vi "Mask From Contour.vi"(0 "Contour":T1, 1 "Size":T2, 5 "error in (no error)":errorcluster) -> (14 "image out":refnum<class "MSC Image.lvclass">, 15 "contourAreaPixel":dbl, 16 "contourLengthPixel":dbl, 17 "Bounding Box":T1, 19 "error out":errorcluster)   [LabVIEW 2016, in "MSC Image.lvclass"]
doc: "Calculates a mask image from a contour. Each pixel within the contour is marked."
uses:
  MSC Image.lvclass
  Dependencies/x86/MSC I Process32.dll
  controls/Image Type.ctl
  controls/Contour.ctl
  controls/Size.ctl
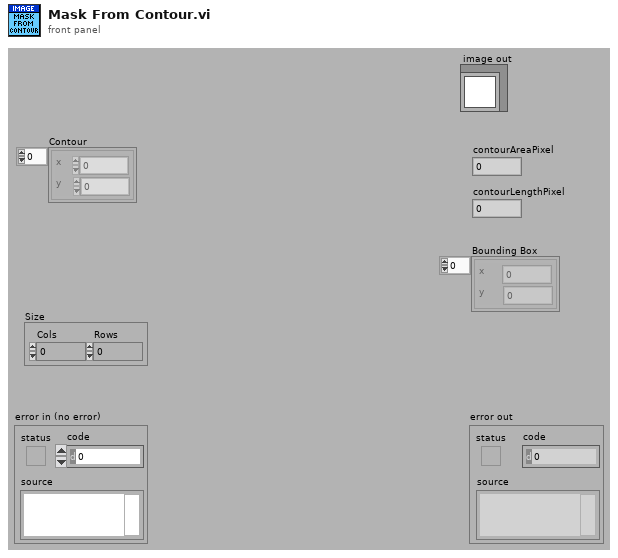
[diagram p1: front panel]
types:
  T1 = typedef "MSC Image.lvclass/Contour.ctl" = cluster{"x":i16, "y":i16}[]
  T2 = typedef "MSC Image.lvclass/Size.ctl" = cluster{"Cols":i32, "Rows":i32}
  T3 = typedef "MSC Image.lvclass/Image Type.ctl" = i32
  T4 = typedef "Image.ctl" = cluster{"Pointer":u64, "Size":T5, "Image Type":T6, "Time Stamp":timestamp, "Variant":variant}
  T5 = typedef "Size.ctl" = cluster{"Cols":i32, "Rows":i32}
  T6 = typedef "Image Type.ctl" = i32
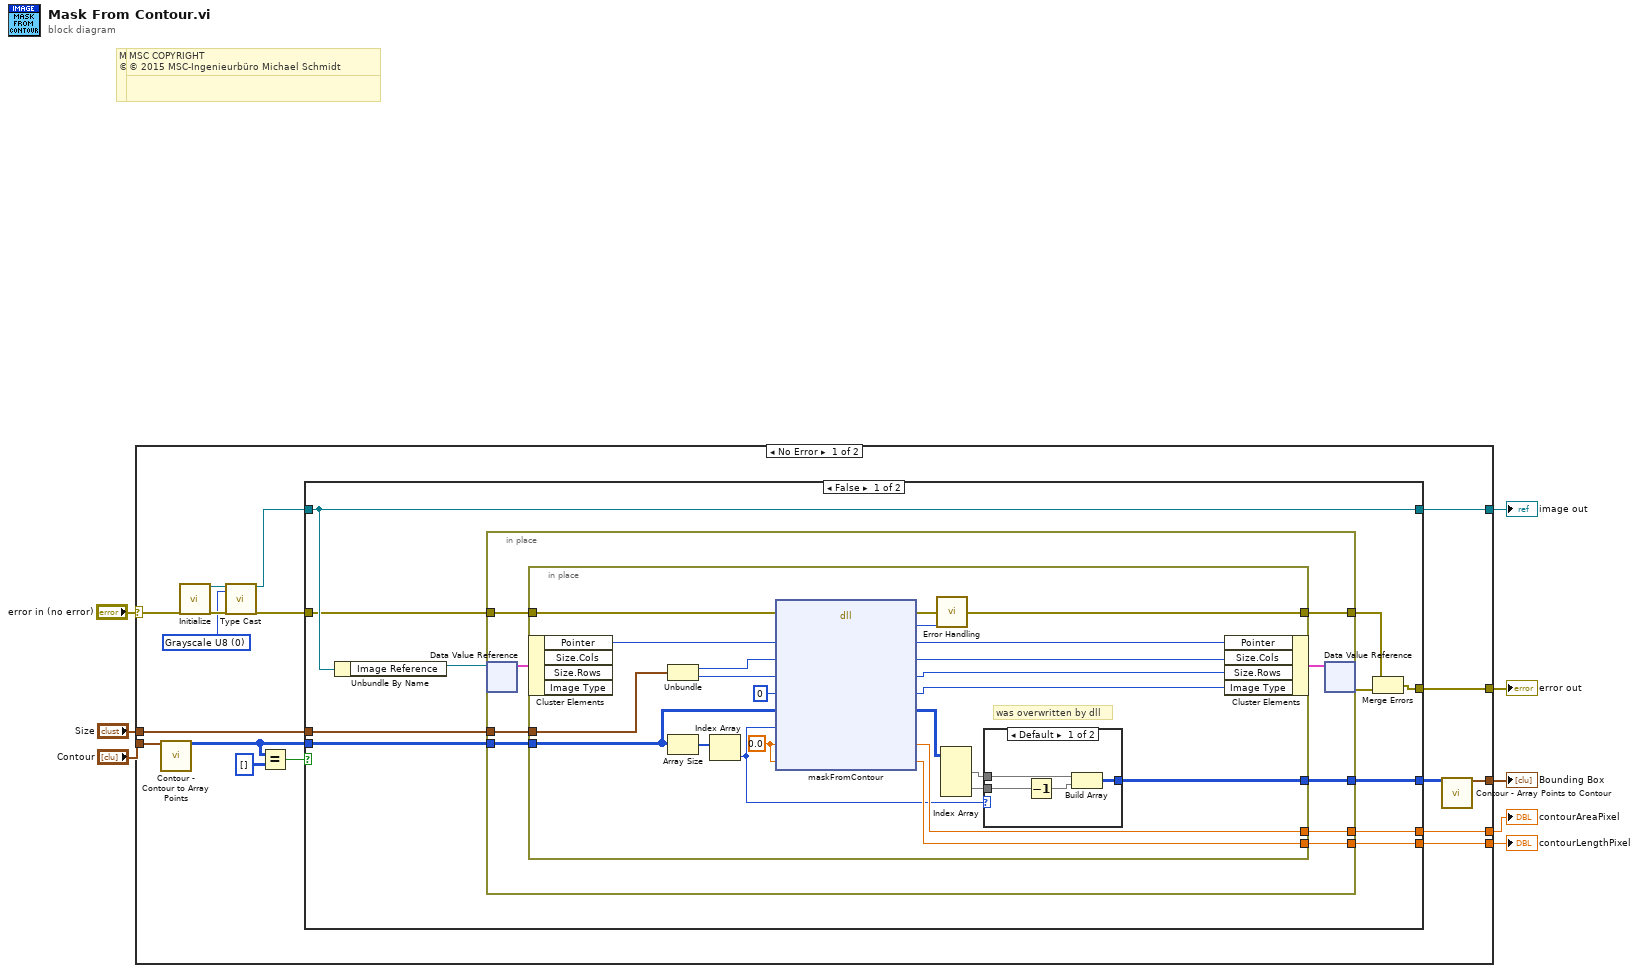
[diagram p0: block diagram]
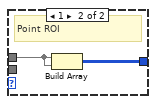
[diagram p2: hidden frame]
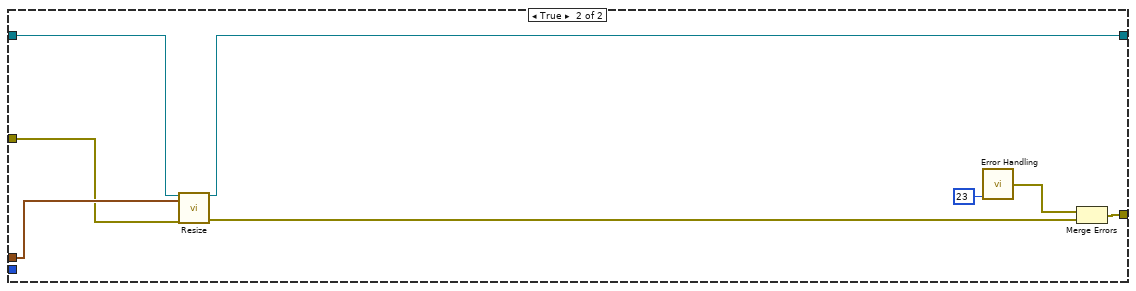
[diagram p3: hidden frame]
diagram:
  # "MSC COPYRIGHT\n© 2016 MSC-Ingenieurbüro Michael Schmidt"
  # "MSC COPYRIGHT\n© 2016 MSC-Ingenieurbüro Michael Schmidt"
  # "MSC COPYRIGHT\n© 2015 MSC-Ingenieurbüro Michael Schmidt"
  # "MSC COPYRIGHT\n© 2015 MSC-Ingenieurbüro Michael Schmidt"
  n1 = case shown="No Error" "error in (no error)" {
    selector: "error in (no error)" -> [w14 w83]
    tunnel: [w24 w83] -> w2
    tunnel: [w25 _] -> w3
    tunnel: "Contour" -> [w18 _]
    tunnel: [w23 _] -> w8
    tunnel: [w22 _] -> w7
    tunnel: [w15 _] -> w4
    tunnel: "Size" -> [w21 _]
    frame No Error {
      w9 = T3 0 items=["Grayscale U8"=0, "Grayscale U16"=2, "Grayscale Single"=5, "Grayscale Double"=6, "RGB U8"=16] ("Image Type")
      n2 = call "Contour - Contour to Array Points.vi"("Contour"=w18) -> ("Array Points"=w17:i16[][])  [unwired: 14 in]
      n3 = call "Initialize.vi"("error in (no error)"=w14) -> ("image out"=w13:refnum<class "MSC Image.lvclass">, "error out"=w11:errorcluster)  [unwired: 17 in]
      n4 = call-dynamic "Type Cast.vi"("image in"=w13, "Image Type"=w9, "error in (no error)"=w11) -> ("image out"=w12:refnum<class "MSC Image.lvclass">, "error out"=w10:errorcluster)  [unwired: 15 in]
      n5 = Equal?(x=w17, y=i32[][] []) -> (x = y?=w19:bool)
      n6 = case shown="False" w19 {
        tunnel: w12 -> [w27 w80]
        tunnel: [w27 w79] -> w25
        tunnel: [w34 w82] -> w24
        tunnel: w10 -> [w26 w78]
        tunnel: w17 -> [w33 _]
        tunnel: [w32 _] -> w23
        tunnel: [w31 _] -> w22
        tunnel: [w30 _] -> w16
        tunnel: w21 -> [w29 w81]
        frame False {
          n7 = Unbundle By Name(w27) -> ("Image Reference"=w28:refnum<data-value>)
          n8 = in-place {
            in-place-border: w26 -> [w43]
            in-place-border: [w42] -> w35
            in-place-border: w33 -> [w41]
            in-place-border: [w40] -> w32
            in-place-border: [w39] -> w31
            in-place-border: [w38] -> w30
            in-place-border: w29 -> [w37]
            n9 = in-place-dvr #1(w28) -> (w44:T4)  [unwired: 1 out]
            n10 = in-place {
              in-place-border: w43 -> [w47]
              in-place-border: [w68] -> w42
              in-place-border: w41 -> [w51]
              in-place-border: [w59] -> w40
              in-place-border: [w58] -> w39
              in-place-border: [w48] -> w38
              in-place-border: w37 -> [w56]
              w60 = 0.0 ("contourAreaPixel")
              # "was overwritten by dll"
              n11 = in-place-cluster #2(w44) -> ("Pointer"=w65:u64)  [unwired: 3 out]
              n12 = Unbundle(w56) -> ("Cols"=w55:i32, "Rows"=w54:i32)
              n13 = Array Size(array=w51) -> (size(s)=w53:i32[])
              n14 = Index Array(array=w53) -> (element=w52:i32)  [unwired: 1 in]
              n15 = dll-call lib="C:/Users/MSC/LabVIEW Projekte/LV 2014/MSC I-Process/user.lib/MSC-I Process/Dependencies/x86/MSC I Process*.dll" fn="maskFromContour"(error in=w47, "pointer"=w65, "cols"=w55, "rows"=w54, "type"=0, "points"=w51, "pointsAmount"=w52, "contourAreaPixel"=w60, "contourLengthPixel"=w60) -> (error out=w67:errorcluster, "error"=w66:i32, "pointer"=w64:u64, "cols"=w63:i32, "rows"=w62:i32, "type"=w61:i32, "points"=w57:i32[][], "contourAreaPixel"=w58:dbl, "contourLengthPixel"=w59:dbl)  [unwired: 3 in, 1 out]
              n16 = call "Error Handling.vi"("error in (no error)"=w67, "return type"=w66) -> ("error out"=w68:errorcluster)  [unwired: 12 in, 1 out]
              n17 = Index Array(array=w57) -> (element #1=w50:i32[], element #2=w49:i32[])  [unwired: 4 in]
              n18 = case shown="Default" w52 {
                tunnel: w50 -> [w71 w74]
                tunnel: w49 -> [w70 _]
                tunnel: [w69 w73] -> w48
                frame Default {
                  n19 = Decrement(x=w70) -> (x-1=w72:i32[])
                  n20 = Build Array(w71, w72) -> (w69:i32[][])
                }
                frame 1 {
                  # "Point ROI"
                  n21 = Build Array(w74, w74) -> (w73:i32[][])
                }
              }
              n22 = in-place-cluster #2("Pointer"=w64, "Size.Cols"=w63, "Size.Rows"=w62, "Image Type"=w61) -> (w45:T4)
            }
            n23 = in-place-dvr #1(w45) -> (w36:errorcluster)  [unwired: 1 out]
          }
          n24 = Merge Errors(w35, w36) -> (w34:errorcluster)
        }
        frame True {
          n25 = call-dynamic "Resize.vi"("image in"=w80, "Size"=w81, "error in (no error)"=w78) -> ("image out"=w79:refnum<class "MSC Image.lvclass">, "error out"=w77:errorcluster)  [unwired: 15 in]
          n26 = call "Error Handling.vi"("return type"=23) -> ("error out"=w75:errorcluster)  [unwired: 13 in, 1 out]
          n27 = Merge Errors(w75, w77) -> (w82:errorcluster)
        }
      }
      n28 = call "Contour - Array Points to Contour.vi"("Array Points"=w16) -> ("Contour"=w15:T1)  [unwired: 14 in]
    }
    frame Error {
    }
  }
  "error out" <- w2
  "image out" <- w3
  "contourAreaPixel" <- w7
  "contourLengthPixel" <- w8
  "Bounding Box" <- w4
